vi "DoNanoCmdSimple.vi"(4 "Pin 2":u32, 5 "SerialNotOpen?":bool, 6 "Wait after response":bool=TRUE, 7 "error in (no error)":errorcluster, 8 "Pin 1":u32, 9 "Nano Op":T1=enum."Get analog pin voltage", 10 "VISA resource name":refnum<visa-resource-name>="COM20") -> (0 "error out":errorcluster={"status"=FALSE, "code"=1073676294, "source"="VISA Read in DoNanoCmd.vi"}, 1 "Response length":i32, 2 "Read Value":dbl, 3 "VISA resource name 2":refnum<visa-resource-name>="COM20")   [LabVIEW 2013]
uses:
  NanoCmds.ctl
  Test Globals/Global 1.vi
panel:
  out "return count":u32
  out "timeout":bool
  in  "WaitForResponse":string
  out "read buffer":string
  in  "Relay Control Port":u32
  in  "Sense Resistor":dbl
  in  "Current Limit":dbl
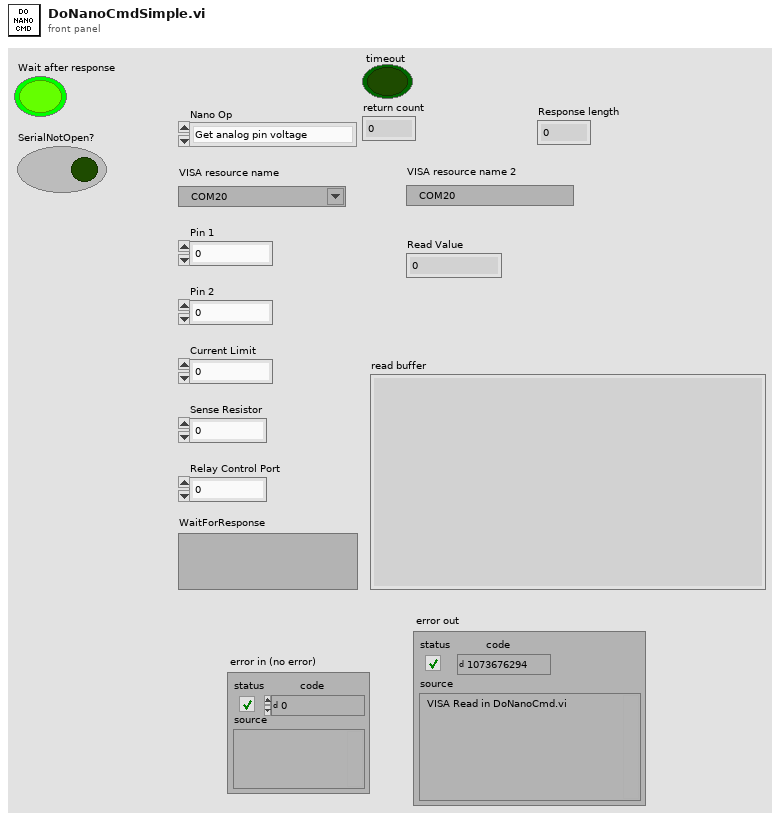
[diagram p1: front panel]
types:
  T1 = typedef "NanoCmds.ctl" = enum16{"Make digital port an output", "Make digital port an input", "Set digital pin high", "Set digital pin low", "Get digital pin state", "Get analog pin voltage", "Get analog pins difference", "Get ohms at analog pin", "Turn on current limit", "Reset Nano device", "Get digital pin state pullup", "Read current", "Initialize", "Power up uut", "Power down uut", "Get uut current draw", "Set ADC volts high", "Set ADC volts low", "Start up uut modem", "Get CTS state", "Get on_nsleep state", "Reset modem", "Get lid state", "Wait for lid closed", "Wait for lid open", "Power up, start, get curr", "Check if X2 shorted", "Power up and start up", "Check X3 shorted", "Get RTS state", "Get DTR state", "Reboot 1002759"}
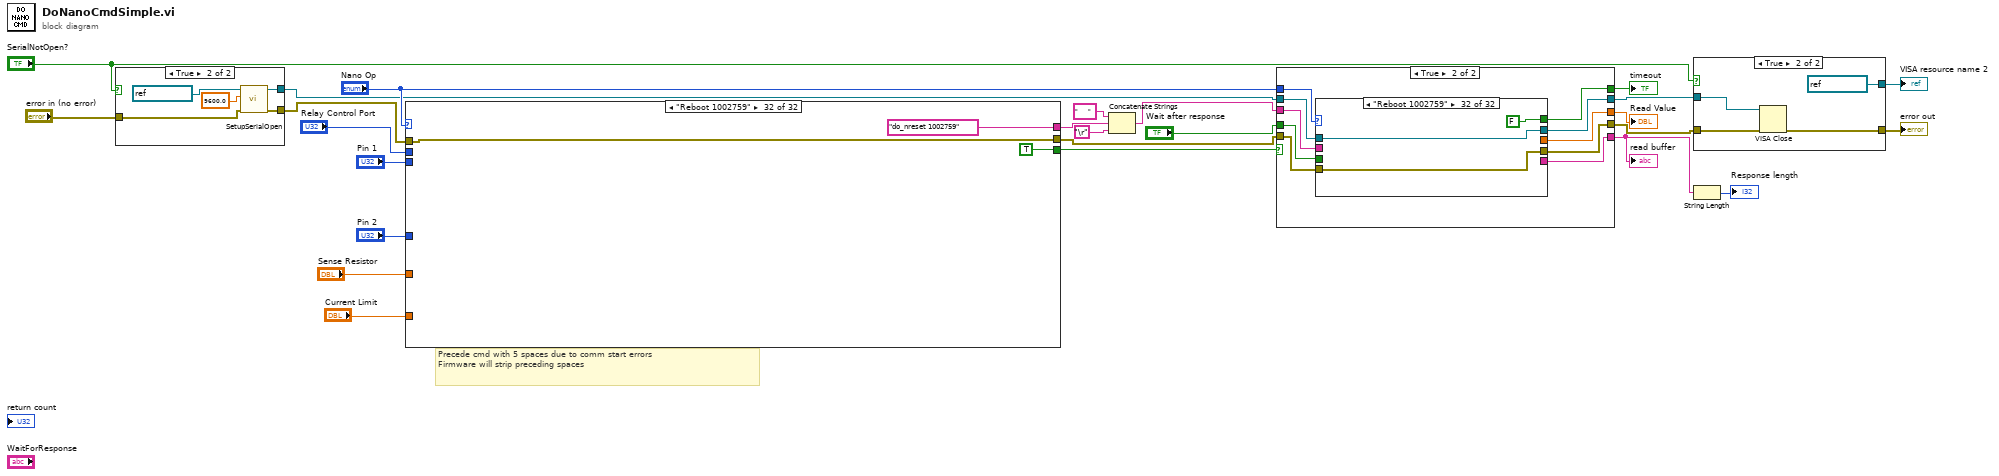
[diagram p0: block diagram]
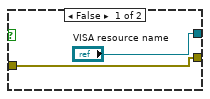
[diagram p3: hidden frame]
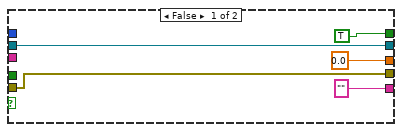
[diagram p4: hidden frame]
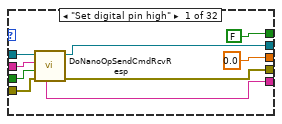
[diagram p5: hidden frame]
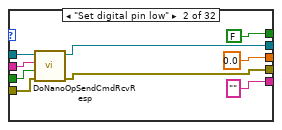
[diagram p6: hidden frame]
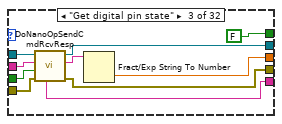
[diagram p7: hidden frame]
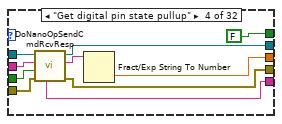
[diagram p8: hidden frame]
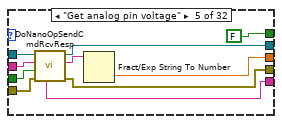
[diagram p9: hidden frame]
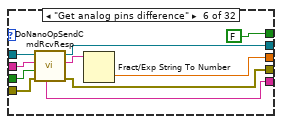
[diagram p10: hidden frame]
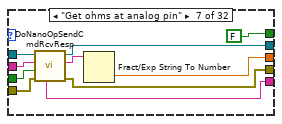
[diagram p11: hidden frame]
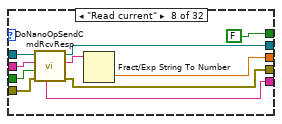
[diagram p12: hidden frame]
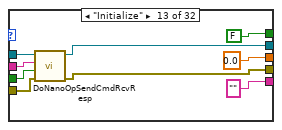
[diagram p17: hidden frame]
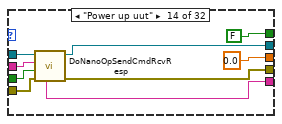
[diagram p18: hidden frame]
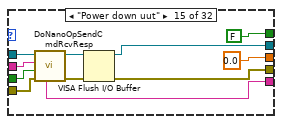
[diagram p19: hidden frame]
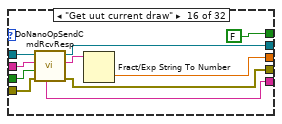
[diagram p20: hidden frame]
diagram:
  # "Precede cmd with 5 spaces due to comm start errors\nFirmware will strip preceding spaces"
  n1 = case shown="True" "SerialNotOpen?" {
    tunnel: ["VISA resource name" w29] -> w13
    tunnel: "error in (no error)" -> [w26 w32]
    tunnel: [w26 w28] -> w7
    frame False {
    }
    frame True {
      n2 = call "SetupSerialOpen.vi"("error in (no error)"=w32, "Baud"=9600.0, "VISA Refnum in"=refnum<visa-resource-name> "COM21") -> ("error out"=w28:errorcluster, "VISA session"=w29:refnum<visa-resource-name>)  [unwired: 7 in]
    }
  }
  n3 = case shown="\"Reboot 1002759\"" "Nano Op" {
    tunnel: w7 -> [w38 w47 w50 w69 w86 w103 w117 w127 w141 _ w167 _ _ w172 w175 w178 w181 w184 w187 w190 w193 w196 w199 w201 w204 w216 w231 w237 w240 w243 w246 w248]
    tunnel: [w38 w47 w49 w68 w85 w102 w117 w127 w141 _ w169 _ _ w172 w175 w178 w181 w184 w187 w190 w193 w196 w199 w201 w204 w216 w231 w237 w240 w243 w246 w248] -> w15
    tunnel: "Pin 1" -> [w36 _ w53 w70 w87 w104 w122 w128 w142 w159 _ _ _ _ _ _ _ _ _ _ _ _ _ _ _ _ _ _ _ _ _ _]
    tunnel: [w39 "INIT" w56 w73 w90 w107 w121 w131 w145 w161 _ _ _ "power_up" "power_down" "curr" "adc_hi" "adc_low" "start_up" "cts" "on_nsleep" "" "lid" "WAITLIDCLOSED" "WAITLIDOPEN" w217 w232 "x2_shorted" "x3_shorted" "read_rts" "read_dtr" "do_nreset 1002759"] -> w18
    tunnel: "Pin 2" -> [_ _ _ _ _ _ w119 _ _ w158 _ _ _ _ _ _ _ _ _ _ _ _ _ _ _ _ _ _ _ _ _ _]
    tunnel: "Relay Control Port" -> [_ _ _ _ _ _ _ _ _ w160 _ _ _ _ _ _ _ _ _ _ _ _ _ _ _ _ _ _ _ _ _ _]
    tunnel: "Sense Resistor" -> [_ _ _ _ _ _ _ _ _ w155 _ _ _ _ _ _ _ _ _ _ _ _ _ _ _ _ _ _ _ _ _ _]
    tunnel: "Current Limit" -> [_ _ _ _ _ _ _ _ _ w154 _ _ _ _ _ _ _ _ _ _ _ _ _ _ _ _ _ _ _ _ _ _]
    tunnel: [w33 _ w51 w66 w83 w100 _ w125 w139 _ _ _ _ TRUE TRUE TRUE TRUE TRUE TRUE TRUE TRUE FALSE TRUE TRUE TRUE TRUE TRUE TRUE TRUE TRUE TRUE TRUE] -> w12
    frame "Set digital pin high" {
      n4 = In Range and Coerce(upper limit=u32 19, x=w36, lower limit=u32 2) -> (In Range?=w37:bool)  [unwired: 1 out]
      n5 = case shown="True" w37 {
        selector: w37 -> [w40 w41]
        tunnel: w36 -> [_ w43]
        tunnel: [_ w42] -> w39
        tunnel: [w40 w41] -> w33
        frame False {
        }
        frame True {
          n6 = Number To Decimal String(number=w43) -> (decimal integer string=w44:string)  [unwired: 1 in]
          n7 = Concatenate Strings("DIG_HI", "," ("string"), w44) -> (w42:string)
        }
      }
    }
    frame "Initialize" {
    }
    frame "Set digital pin low" {
      n8 = In Range and Coerce(upper limit=u32 19, x=w53, lower limit=u32 2) -> (In Range?=w52:bool)  [unwired: 1 out]
      n9 = case shown="True" w52 {
        selector: w52 -> [w58 w60]
        tunnel: [_ w62] -> w56
        tunnel: w53 -> [_ w61]
        tunnel: [w58 w60] -> w51
        tunnel: w50 -> [w57 w59]
        tunnel: [w57 w59] -> w49
        frame False {
        }
        frame True {
          n10 = Number To Decimal String(number=w61) -> (decimal integer string=w63:string)  [unwired: 1 in]
          n11 = Concatenate Strings("DIG_LO", "," ("string"), w63) -> (w62:string)
        }
      }
    }
    frame "Get digital pin state" {
      n12 = In Range and Coerce(upper limit=u32 19, x=w70, lower limit=u32 2) -> (In Range?=w67:bool)  [unwired: 1 out]
      n13 = case shown="True" w67 {
        selector: w67 -> [w75 w76]
        tunnel: [_ w79] -> w73
        tunnel: w70 -> [_ w78]
        tunnel: w69 -> [w74 w77]
        tunnel: [w74 w77] -> w68
        tunnel: [w75 w76] -> w66
        frame False {
        }
        frame True {
          n14 = Number To Decimal String(number=w78) -> (decimal integer string=w80:string)  [unwired: 1 in]
          n15 = Concatenate Strings("DIG_STATE", "," ("string"), w80) -> (w79:string)
        }
      }
    }
    frame "Get digital pin state pullup" {
      n16 = In Range and Coerce(upper limit=u32 13, x=w87, lower limit=u32 2) -> (In Range?=w84:bool)  [unwired: 1 out]
      n17 = case shown="True" w84 {
        selector: w84 -> [w92 w94]
        tunnel: [_ w93] -> w90
        tunnel: w87 -> [_ w96]
        tunnel: w86 -> [w91 w95]
        tunnel: [w91 w95] -> w85
        tunnel: [w92 w94] -> w83
        frame False {
        }
        frame True {
          n18 = Number To Decimal String(number=w96) -> (decimal integer string=w97:string)  [unwired: 1 in]
          n19 = Concatenate Strings("DIG_STATE_PULLUP", "," ("string"), w97) -> (w93:string)
        }
      }
    }
    frame "Get analog pin voltage" {
      n20 = In Range and Coerce(upper limit=u32 5, x=w104, lower limit=u32 0) -> (In Range?=w101:bool)  [unwired: 1 out]
      n21 = case shown="True" w101 {
        selector: w101 -> [w109 w110]
        tunnel: [_ w113] -> w107
        tunnel: w104 -> [_ w112]
        tunnel: w103 -> [w108 w111]
        tunnel: [w108 w111] -> w102
        tunnel: [w109 w110] -> w100
        frame False {
        }
        frame True {
          n22 = Number To Decimal String(number=w112) -> (decimal integer string=w114:string)  [unwired: 1 in]
          n23 = Concatenate Strings("ANA_READ", "," ("string"), w114) -> (w113:string)
        }
      }
    }
    frame "Get analog pins difference" {
      w120 = "," ("string")
      n24 = Number To Decimal String(number=w122) -> (decimal integer string=w123:string)  [unwired: 1 in]
      n25 = Number To Decimal String(number=w119) -> (decimal integer string=w118:string)  [unwired: 1 in]
      n26 = Concatenate Strings("ANA_DIF", w120, w123, w120, w118) -> (w121:string)
    }
    frame "Get ohms at analog pin" {
      n27 = In Range and Coerce(upper limit=u32 5, x=w128, lower limit=u32 0) -> (In Range?=w126:bool)  [unwired: 1 out]
      n28 = case shown="True" w126 {
        selector: w126 -> [w132 w133]
        tunnel: [_ w135] -> w131
        tunnel: w128 -> [_ w134]
        tunnel: [w132 w133] -> w125
        frame False {
        }
        frame True {
          n29 = Number To Decimal String(number=w134) -> (decimal integer string=w136:string)  [unwired: 1 in]
          n30 = Concatenate Strings("GET_OHMS", "," ("string"), w136) -> (w135:string)
        }
      }
    }
    frame "Read current" {
      n31 = In Range and Coerce(upper limit=u32 5, x=w142, lower limit=u32 0) -> (In Range?=w140:bool)  [unwired: 1 out]
      n32 = case shown="True" w140 {
        selector: w140 -> [w146 w147]
        tunnel: [_ w149] -> w145
        tunnel: w142 -> [_ w148]
        tunnel: [w146 w147] -> w139
        frame False {
        }
        frame True {
          n33 = Number To Decimal String(number=w148) -> (decimal integer string=w150:string)  [unwired: 1 in]
          n34 = Concatenate Strings("READ_CURR", "," ("string"), w150) -> (w149:string)
        }
      }
    }
    frame "Turn on current limit" {
      w153 = i16 3 ("precision (6)")
      w162 = "," ("string")
      n35 = Number To Fractional String(number=w155, precision (6)=w153) -> (F-format string=w157:string)  [unwired: 2 in]
      n36 = Number To Fractional String(number=w154, precision (6)=w153) -> (F-format string=w156:string)  [unwired: 2 in]
      n37 = Number To Decimal String(number=w160) -> (decimal integer string=w165:string)  [unwired: 1 in]
      n38 = Number To Decimal String(number=w159) -> (decimal integer string=w164:string)  [unwired: 1 in]
      n39 = Number To Decimal String(number=w158) -> (decimal integer string=w163:string)  [unwired: 1 in]
      n40 = Concatenate Strings("CURR_LIMIT", w162, w165, w162, w164, w162, w163, w162, w157, w162, w156) -> (w161:string)
    }
    frame "Reset Nano device" {
      n41 = call "WaitMsecs.vi"("error in (no error)"=w167, "Wait Msecs"=1500.0) -> ("error out"=w169:errorcluster)  [unwired: 9 in]
    }
    frame "Make digital port an output" {
    }
    frame "Make digital port an input" {
    }
    frame "Power up uut" {
    }
    frame "Power down uut" {
    }
    frame "Get uut current draw" {
    }
    frame "Set ADC volts high" {
    }
    frame "Set ADC volts low" {
    }
    frame "Start up uut modem" {
    }
    frame "Get CTS state" {
    }
    frame "Get on_nsleep state" {
    }
    frame "Reset modem" {
    }
    frame "Get lid state" {
    }
    frame "Wait for lid closed" {
    }
    frame "Wait for lid open" {
    }
    frame "Power up, start, get curr" {
      n42 = global read "Global 1.vi" "Modem Make"() -> (w209:string)
      n43 = Equal?(x=w209, y="wnc") -> (x = y?=w207:bool)
      n44 = Equal?(x=w209, y="sequans") -> (x = y?=w208:bool)
      n45 = Or(x=w207, y=w208) -> (x .or. y?=w206:bool)
      n46 = global read "Global 1.vi" "reset delay"() -> (w219:u32)
      n47 = Select(t=",9999" ("string"), s=w206, f=",3000" ("string")) -> (s? t:f=w211:string)
      n48 = Number To Decimal String(number=w219) -> (decimal integer string=w218:string)  [unwired: 1 in]
      n49 = Concatenate Strings("pstart_getcurr," ("string"), w218, w211) -> (w217:string)
    }
    frame "Power up and start up" {
      n50 = global read "Global 1.vi" "Modem Make"() -> (w224:string)
      n51 = Equal?(x=w224, y="wnc") -> (x = y?=w222:bool)
      n52 = Equal?(x=w224, y="sequans") -> (x = y?=w223:bool)
      n53 = Or(x=w222, y=w223) -> (x .or. y?=w221:bool)
      n54 = global read "Global 1.vi" "reset delay"() -> (w234:u32)
      n55 = Select(t=",9999" ("string"), s=w221, f=",3000" ("string")) -> (s? t:f=w226:string)
      n56 = Number To Decimal String(number=w234) -> (decimal integer string=w233:string)  [unwired: 1 in]
      n57 = Concatenate Strings("pstart," ("string"), w233, w226) -> (w232:string)
    }
    frame "Check if X2 shorted" {
    }
    frame "Check X3 shorted" {
    }
    frame "Get RTS state" {
    }
    frame "Get DTR state" {
    }
    frame "Reboot 1002759" {
    }
  }
  n58 = Concatenate Strings("     " ("string"), w18, "\r") -> (w16:string)
  n59 = case shown="True" w12 {
    tunnel: "Nano Op" -> [_ w265]
    tunnel: [0.0 w264] -> w19
    tunnel: w16 -> [_ w263]
    tunnel: w15 -> [w254 w262]
    tunnel: ["" ("read buffer") w261] -> w10
    tunnel: [TRUE ("timeout") w260] -> w14
    tunnel: [w254 w259] -> w5
    tunnel: w13 -> [w255 w258]
    tunnel: [w255 w257] -> w4
    tunnel: "Wait after response" -> [_ w256]
    frame False {
    }
    frame True {
      n60 = case shown="\"Reboot 1002759\"" w265 {
        tunnel: w258 -> [w271 w279 w289 w299 w309 w319 w329 w339 w345 w347 w350 w352 w356 w367 w376 w387 w396 w406 w415 w424 w434 w440 w447 w457 w466 w474 w483 w488 w501 w516 w526 w534]
        tunnel: w262 -> [w272 w281 w291 w301 w311 w321 w331 w341 w344 w348 w349 w351 w358 w369 w378 w389 w398 w408 w417 w426 w436 w441 w449 w459 w468 w476 w485 w490 w503 w513 w523 w535]
        tunnel: [w268 w277 w286 w297 w307 w318 w328 w337 w344 w348 w349 w351 w355 w365 w380 w385 w394 w404 w413 w422 w432 w441 w445 w456 w464 w471 w481 w494 w507 w518 w528 w535] -> w259
        tunnel: [0.0 0.0 w293 w303 w313 w323 w333 w343 _ _ _ _ 0.0 0.0 0.0 w391 0.0 0.0 0.0 w428 w438 _ w451 0.0 0.0 w478 0.0 ("f") w493 w506 w519 w529 _] -> w264
        tunnel: w263 -> [w270 w280 w290 w300 w310 w320 w330 w340 _ w346 _ _ w357 w368 w377 w388 w397 w407 w416 w425 w435 _ w448 w458 w467 w475 w484 w487 w500 w515 w525 _]
        tunnel: [w269 "" ("read buffer") w285 w295 w306 w315 w326 w338 _ w346 _ _ "" ("read buffer") w364 w372 w383 w393 w403 w412 w420 w430 _ w444 w453 w462 _ _ _ _ w517 w527 _] -> w261
        tunnel: [FALSE ("timeout") FALSE ("timeout") FALSE ("timeout") FALSE ("timeout") FALSE ("timeout") FALSE ("timeout") FALSE ("timeout") FALSE ("timeout") _ _ _ _ FALSE ("timeout") FALSE ("timeout") FALSE ("timeout") FALSE ("timeout") FALSE ("timeout") FALSE ("timeout") FALSE ("timeout") FALSE ("timeout") FALSE ("timeout") FALSE ("timeout") FALSE ("timeout") FALSE ("timeout") FALSE ("timeout") FALSE ("timeout") FALSE ("timeout") FALSE ("timeout") FALSE ("timeout") FALSE ("timeout") FALSE ("timeout") FALSE ("timeout")] -> w260
        tunnel: [w267 w276 w288 w296 w308 w317 w325 w335 w345 w347 w350 w352 w354 w366 w381 w386 w395 w405 w414 w423 w433 w440 w446 w455 w465 w472 w482 w492 w505 w520 w530 w534] -> w257
        tunnel: w256 -> [w266 w275 w284 w294 w304 w314 w324 w334 _ _ _ _ w353 w362 w371 w382 w392 w401 w410 w419 w429 _ w442 w452 w461 w470 w480 w489 w502 w514 w524 _]
        frame "Set digital pin high" {
          n61 = call "DoNanoOpSendCmdRcvResp.vi"("error in (no error)"=w272, "Wait after response"=w266, "Cmd String"=w270, "VISA resource name"=w271) -> ("error out"=w268:errorcluster, "VISA resource name out"=w267:refnum<visa-resource-name>, "read buffer"=w269:string)  [unwired: 1 in, 4 out]
        }
        frame "Set digital pin low" {
          n62 = call "DoNanoOpSendCmdRcvResp.vi"("error in (no error)"=w281, "Wait after response"=w275, "Cmd String"=w280, "VISA resource name"=w279) -> ("error out"=w277:errorcluster, "VISA resource name out"=w276:refnum<visa-resource-name>)  [unwired: 1 in, 5 out]
        }
        frame "Get digital pin state" {
          n63 = call "DoNanoOpSendCmdRcvResp.vi"("error in (no error)"=w291, "Wait after response"=w284, "Cmd String"=w290, "VISA resource name"=w289) -> ("error out"=w286:errorcluster, "Line 1"=w287:string, "VISA resource name out"=w288:refnum<visa-resource-name>, "read buffer"=w285:string)  [unwired: 1 in, 3 out]
          n64 = Fract/Exp String To Number(string=w287) -> (number=w293:dbl)  [unwired: 3 in, 1 out]
        }
        frame "Get digital pin state pullup" {
          n65 = call "DoNanoOpSendCmdRcvResp.vi"("error in (no error)"=w301, "Wait after response"=w294, "Cmd String"=w300, "VISA resource name"=w299) -> ("error out"=w297:errorcluster, "Line 1"=w298:string, "VISA resource name out"=w296:refnum<visa-resource-name>, "read buffer"=w295:string)  [unwired: 1 in, 3 out]
          n66 = Fract/Exp String To Number(string=w298) -> (number=w303:dbl)  [unwired: 3 in, 1 out]
        }
        frame "Get analog pin voltage" {
          n67 = call "DoNanoOpSendCmdRcvResp.vi"("error in (no error)"=w311, "Wait after response"=w304, "Cmd String"=w310, "VISA resource name"=w309) -> ("error out"=w307:errorcluster, "Line 1"=w305:string, "VISA resource name out"=w308:refnum<visa-resource-name>, "read buffer"=w306:string)  [unwired: 1 in, 3 out]
          n68 = Fract/Exp String To Number(string=w305) -> (number=w313:dbl)  [unwired: 3 in, 1 out]
        }
        frame "Get analog pins difference" {
          n69 = call "DoNanoOpSendCmdRcvResp.vi"("error in (no error)"=w321, "Wait after response"=w314, "Cmd String"=w320, "VISA resource name"=w319) -> ("error out"=w318:errorcluster, "Line 1"=w316:string, "VISA resource name out"=w317:refnum<visa-resource-name>, "read buffer"=w315:string)  [unwired: 1 in, 3 out]
          n70 = Fract/Exp String To Number(string=w316) -> (number=w323:dbl)  [unwired: 3 in, 1 out]
        }
        frame "Get ohms at analog pin" {
          n71 = call "DoNanoOpSendCmdRcvResp.vi"("error in (no error)"=w331, "Wait after response"=w324, "Cmd String"=w330, "VISA resource name"=w329) -> ("error out"=w328:errorcluster, "Line 1"=w327:string, "VISA resource name out"=w325:refnum<visa-resource-name>, "read buffer"=w326:string)  [unwired: 1 in, 3 out]
          n72 = Fract/Exp String To Number(string=w327) -> (number=w333:dbl)  [unwired: 3 in, 1 out]
        }
        frame "Read current" {
          n73 = call "DoNanoOpSendCmdRcvResp.vi"("error in (no error)"=w341, "Wait after response"=w334, "Cmd String"=w340, "VISA resource name"=w339) -> ("error out"=w337:errorcluster, "Line 1"=w336:string, "VISA resource name out"=w335:refnum<visa-resource-name>, "read buffer"=w338:string)  [unwired: 1 in, 3 out]
          n74 = Fract/Exp String To Number(string=w336) -> (number=w343:dbl)  [unwired: 3 in, 1 out]
        }
        frame "Turn on current limit" {
        }
        frame "Reset Nano device" {
        }
        frame "Make digital port an output" {
        }
        frame "Make digital port an input" {
        }
        frame "Initialize" {
          n75 = call "DoNanoOpSendCmdRcvResp.vi"("error in (no error)"=w358, "Wait after response"=w353, "Cmd String"=w357, "VISA resource name"=w356) -> ("error out"=w355:errorcluster, "VISA resource name out"=w354:refnum<visa-resource-name>)  [unwired: 1 in, 5 out]
        }
        frame "Power up uut" {
          n76 = call "DoNanoOpSendCmdRcvResp.vi"("error in (no error)"=w369, "Wait after response"=w362, "Cmd String"=w368, "VISA resource name"=w367) -> ("error out"=w365:errorcluster, "VISA resource name out"=w366:refnum<visa-resource-name>, "read buffer"=w364:string)  [unwired: 1 in, 4 out]
        }
        frame "Power down uut" {
          n77 = call "DoNanoOpSendCmdRcvResp.vi"("error in (no error)"=w378, "Wait after response"=w371, "Cmd String"=w377, "VISA resource name"=w376) -> ("error out"=w373:errorcluster, "VISA resource name out"=w375:refnum<visa-resource-name>, "read buffer"=w372:string)  [unwired: 1 in, 4 out]
          n78 = VISA Flush I/O Buffer(VISA resource name=w375, error in (no error)=w373) -> (VISA resource name out=w381:refnum<visa-resource-name>, error out=w380:errorcluster)  [unwired: 1 in]
        }
        frame "Get uut current draw" {
          n79 = call "DoNanoOpSendCmdRcvResp.vi"("error in (no error)"=w389, "Wait after response"=w382, "Cmd String"=w388, "VISA resource name"=w387) -> ("error out"=w385:errorcluster, "Line 1"=w384:string, "VISA resource name out"=w386:refnum<visa-resource-name>, "read buffer"=w383:string)  [unwired: 1 in, 3 out]
          n80 = Fract/Exp String To Number(string=w384) -> (number=w391:dbl)  [unwired: 3 in, 1 out]
        }
        frame "Set ADC volts high" {
          n81 = call "DoNanoOpSendCmdRcvResp.vi"("error in (no error)"=w398, "Wait after response"=w392, "Cmd String"=w397, "VISA resource name"=w396) -> ("error out"=w394:errorcluster, "VISA resource name out"=w395:refnum<visa-resource-name>, "read buffer"=w393:string)  [unwired: 1 in, 4 out]
        }
        frame "Set ADC volts low" {
          n82 = call "DoNanoOpSendCmdRcvResp.vi"("error in (no error)"=w408, "Wait after response"=w401, "Cmd String"=w407, "VISA resource name"=w406) -> ("error out"=w404:errorcluster, "VISA resource name out"=w405:refnum<visa-resource-name>, "read buffer"=w403:string)  [unwired: 1 in, 4 out]
        }
        frame "Start up uut modem" {
          n83 = call "DoNanoOpSendCmdRcvResp.vi"("error in (no error)"=w417, "Wait after response"=w410, "Cmd String"=w416, "VISA resource name"=w415) -> ("error out"=w413:errorcluster, "VISA resource name out"=w414:refnum<visa-resource-name>, "read buffer"=w412:string)  [unwired: 1 in, 4 out]
        }
        frame "Get CTS state" {
          n84 = call "DoNanoOpSendCmdRcvResp.vi"("error in (no error)"=w426, "Wait after response"=w419, "Cmd String"=w425, "VISA resource name"=w424) -> ("error out"=w422:errorcluster, "Line 1"=w421:string, "VISA resource name out"=w423:refnum<visa-resource-name>, "read buffer"=w420:string)  [unwired: 1 in, 3 out]
          n85 = Fract/Exp String To Number(string=w421) -> (number=w428:dbl)  [unwired: 3 in, 1 out]
        }
        frame "Get on_nsleep state" {
          n86 = call "DoNanoOpSendCmdRcvResp.vi"("error in (no error)"=w436, "Wait after response"=w429, "Cmd String"=w435, "VISA resource name"=w434) -> ("error out"=w432:errorcluster, "Line 1"=w431:string, "VISA resource name out"=w433:refnum<visa-resource-name>, "read buffer"=w430:string)  [unwired: 1 in, 3 out]
          n87 = Fract/Exp String To Number(string=w431) -> (number=w438:dbl)  [unwired: 3 in, 1 out]
        }
        frame "Reset modem" {
        }
        frame "Get lid state" {
          n88 = call "DoNanoOpSendCmdRcvResp.vi"("error in (no error)"=w449, "Wait after response"=w442, "Cmd String"=w448, "VISA resource name"=w447) -> ("error out"=w445:errorcluster, "Line 1"=w443:string, "VISA resource name out"=w446:refnum<visa-resource-name>, "read buffer"=w444:string)  [unwired: 1 in, 3 out]
          n89 = Fract/Exp String To Number(string=w443) -> (number=w451:dbl)  [unwired: 3 in, 1 out]
        }
        frame "Wait for lid closed" {
          n90 = call "DoNanoOpSendCmdRcvResp.vi"("error in (no error)"=w459, "Wait after response"=w452, "Cmd String"=w458, "VISA resource name"=w457) -> ("error out"=w456:errorcluster, "VISA resource name out"=w455:refnum<visa-resource-name>, "read buffer"=w453:string)  [unwired: 1 in, 4 out]
        }
        frame "Wait for lid open" {
          n91 = call "DoNanoOpSendCmdRcvResp.vi"("error in (no error)"=w468, "Wait after response"=w461, "Cmd String"=w467, "VISA resource name"=w466) -> ("error out"=w464:errorcluster, "VISA resource name out"=w465:refnum<visa-resource-name>, "read buffer"=w462:string)  [unwired: 1 in, 4 out]
        }
        frame "Power up, start, get curr" {
          n92 = call "DoNanoOpSendCmdRcvResp.vi"("error in (no error)"=w476, "Wait after response"=w470, "Cmd String"=w475, "VISA resource name"=w474) -> ("error out"=w471:errorcluster, "Line 1"=w473:string, "VISA resource name out"=w472:refnum<visa-resource-name>)  [unwired: 1 in, 4 out]
          n93 = Fract/Exp String To Number(string=w473) -> (number=w478:dbl)  [unwired: 3 in, 1 out]
        }
        frame "Power up and start up" {
          n94 = call "DoNanoOpSendCmdRcvResp.vi"("error in (no error)"=w485, "Wait after response"=w480, "Cmd String"=w484, "VISA resource name"=w483) -> ("error out"=w481:errorcluster, "VISA resource name out"=w482:refnum<visa-resource-name>)  [unwired: 1 in, 5 out]
        }
        frame "Check if X2 shorted" {
          n95 = call "DoNanoOpSendCmdRcvResp.vi"("error in (no error)"=w490, "Wait after response"=w489, "Cmd String"=w487, "VISA resource name"=w488) -> ("error out"=w494:errorcluster, "Line 1"=w495:string, "VISA resource name out"=w492:refnum<visa-resource-name>)  [unwired: 1 in, 4 out]
          n96 = Equal?(x=w495, y="YES") -> (x = y?=w497:bool)
          n97 = Select(t=1.0, s=w497, f=0.0) -> (s? t:f=w493:dbl)
        }
        frame "Check X3 shorted" {
          n98 = call "DoNanoOpSendCmdRcvResp.vi"("error in (no error)"=w503, "Wait after response"=w502, "Cmd String"=w500, "VISA resource name"=w501) -> ("error out"=w507:errorcluster, "Line 1"=w508:string, "VISA resource name out"=w505:refnum<visa-resource-name>)  [unwired: 1 in, 4 out]
          n99 = Equal?(x=w508, y="YES") -> (x = y?=w510:bool)
          n100 = Select(t=1.0, s=w510, f=0.0) -> (s? t:f=w506:dbl)
        }
        frame "Get RTS state" {
          n101 = call "DoNanoOpSendCmdRcvResp.vi"("error in (no error)"=w513, "Wait after response"=w514, "Cmd String"=w515, "VISA resource name"=w516) -> ("error out"=w518:errorcluster, "Line 1"=w522:string, "VISA resource name out"=w520:refnum<visa-resource-name>, "read buffer"=w517:string)  [unwired: 1 in, 3 out]
          n102 = Fract/Exp String To Number(string=w522) -> (number=w519:dbl)  [unwired: 3 in, 1 out]
        }
        frame "Get DTR state" {
          n103 = call "DoNanoOpSendCmdRcvResp.vi"("error in (no error)"=w523, "Wait after response"=w524, "Cmd String"=w525, "VISA resource name"=w526) -> ("error out"=w528:errorcluster, "Line 1"=w532:string, "VISA resource name out"=w530:refnum<visa-resource-name>, "read buffer"=w527:string)  [unwired: 1 in, 3 out]
          n104 = Fract/Exp String To Number(string=w532) -> (number=w529:dbl)  [unwired: 3 in, 1 out]
        }
        frame "Reboot 1002759" {
        }
      }
    }
  }
  "Read Value" <- w19
  "read buffer" <- w10
  "timeout" <- w14
  n105 = case shown="True" "SerialNotOpen?" {
    tunnel: [w537 w540] -> w6
    tunnel: w5 -> [w537 w541]
    tunnel: w4 -> [w536 w539]
    tunnel: [w536 refnum<visa-resource-name> "COM21" ("VISA resource name out")] -> w3
    frame False {
    }
    frame True {
      n106 = VISA Close(VISA resource name=w539, error in (no error)=w541) -> (error out=w540:errorcluster)
    }
  }
  "error out" <- w6
  "VISA resource name 2" <- w3
  n107 = String Length(string=w10) -> (length=→"Response length":i32)
